vi "output with direct move.vi"() -> ()   [LabVIEW 2012]
uses:
  <vilib>/rvi/eio/common/nirviEmuTemplateMethod_errors.vi
  <vilib>/eio/EIONode/EIONode.xnode
panel:
  in  "Mod8/AO2":fxp<+/-,20,5>
  in  "Mod8/AO0":fxp<+/-,20,5>
  in  "Mod8/AO1":fxp<+/-,20,5>
  in  "Count(uSec)":u32
  out "Mod1/AI0":fxp<+/-,20,5>
  out "Mod1/AI1":fxp<+/-,20,5>
  out "Mod1/AI2":fxp<+/-,20,5>
  out "Mod1/AI3":fxp<+/-,20,5>
  in  "stop":bool
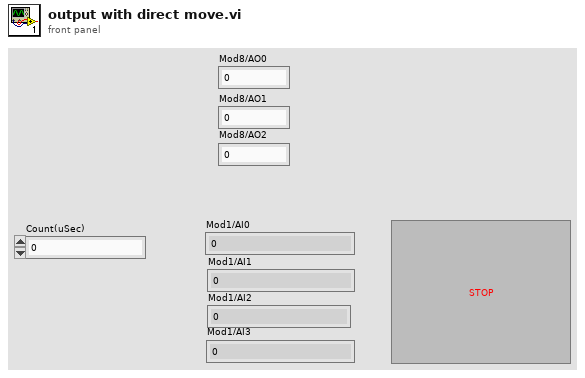
[diagram p1: front panel]
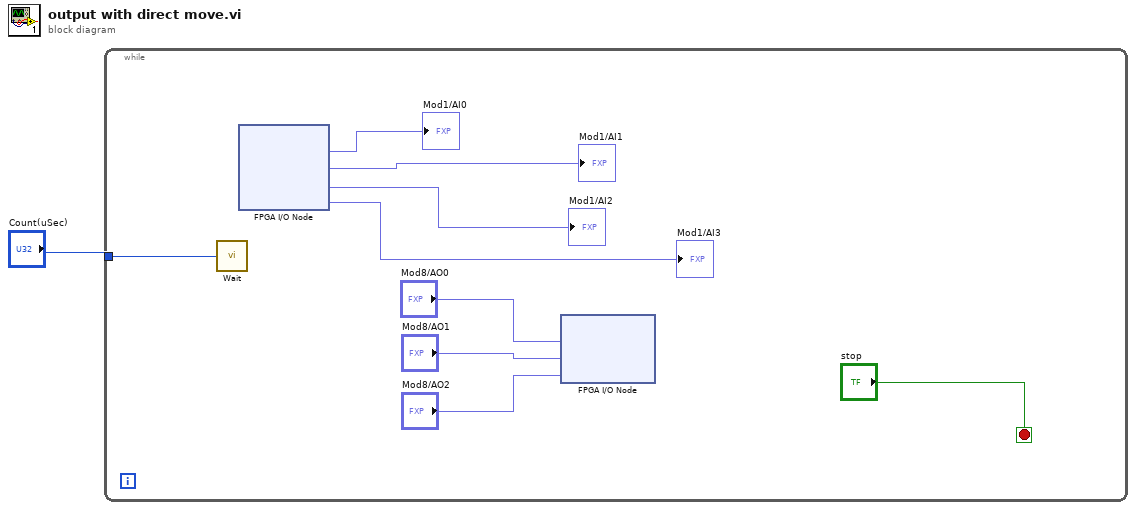
[diagram p0: block diagram]
diagram:
  n1 = while {
    tunnel: "Count(uSec)" -> [w6]
    stop <- "stop" stop-if-true
    n2 = call "Wait"("Count(uSec)"=w6) -> ()  [unwired: 1 out]
    n3 = xnode "FPGA I/O Node"() -> ("Mod1/AI0"=→"Mod1/AI0":fxp<+/-,20,5>, "Mod1/AI1"=→"Mod1/AI1":fxp<+/-,20,5>, "Mod1/AI2"=→"Mod1/AI2":fxp<+/-,20,5>, "Mod1/AI3"=→"Mod1/AI3":fxp<+/-,20,5>)  [unwired: 4 in, 4 out]
    n4 = xnode "FPGA I/O Node"("Mod8/AO0"="Mod8/AO0", "Mod8/AO1"="Mod8/AO1", "Mod8/AO2"="Mod8/AO2") -> ()  [unwired: 3 in, 3 out]
  }
